vi "EJEM16.vi"() -> ()   [LabVIEW 2013]
panel:
  in  "disabled index (col)":i32
  in  "index (row)":i32
  out "size(s)":i32[](array[numeric])
  out "transposed array":dbl[][](array[numeric])
  out "element":dbl
  in  "array":dbl[][](array[numeric])
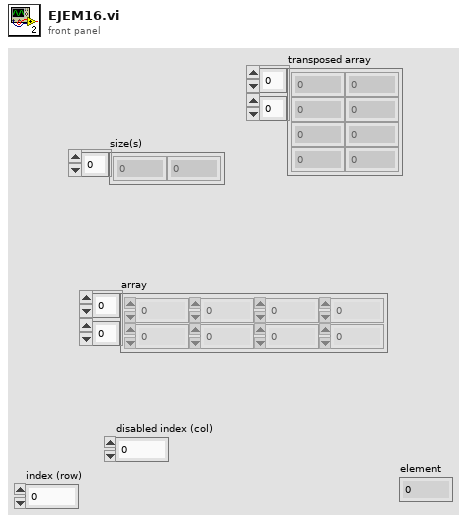
[diagram p1: front panel]
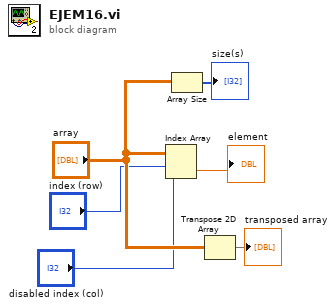
[diagram p0: block diagram]
diagram:
  n1 = Index Array(array="array", index (row)="index (row)", index (col)="disabled index (col)") -> (element=→"element":dbl)
  n2 = Array Size(array="array") -> (size(s)=→"size(s)":i32[])
  n3 = Transpose 2D Array(2D array="array") -> (transposed array=→"transposed array":dbl[][])
